vi "dosimat876_zero.vi"(2 "error in":errorcluster, 3 "Dosimat Port In":refnum<visa-resource-name>="COM1") -> (0 "error out":errorcluster, 1 "Dosimat Port Out":refnum<visa-resource-name>="COM1")   [LabVIEW 2010]
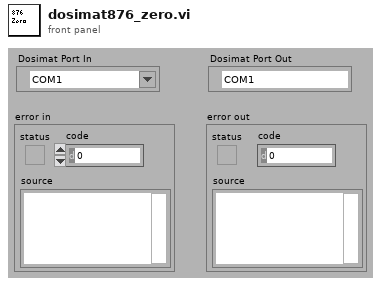
[diagram p1: front panel]
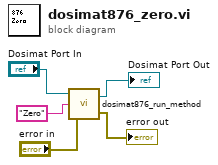
[diagram p0: block diagram]
diagram:
  n1 = call "dosimat876_run_method.vi"("error in"="error in", "Method"="Zero", "Dosimat Port In"="Dosimat Port In") -> ("error out"=→"error out":errorcluster, "Dosimat Port Out"=→"Dosimat Port Out":refnum<visa-resource-name>)
